vi "file header.vi"(8 "error in (no error)":errorcluster, 11 "Keywords Log File in":refnum<class "Keywords Log File.lvclass">) -> (0 "error out":errorcluster, 3 "Keywords Log File out":refnum<class "Keywords Log File.lvclass">)   [LabVIEW 2018, in "Keywords Log File.lvclass"]
uses:
  Keywords Log File.lvclass
  Log File/Log File.lvclass
  C:/Users/Denis/Desktop/S4ACS/S4ACS/Log File/Log File.lvclass
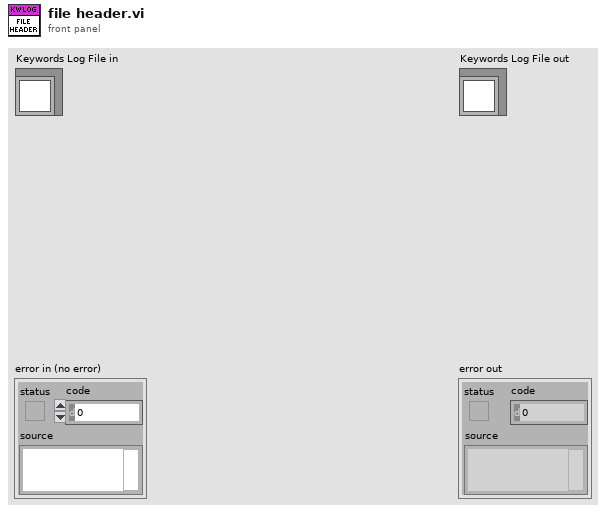
[diagram p1: front panel]
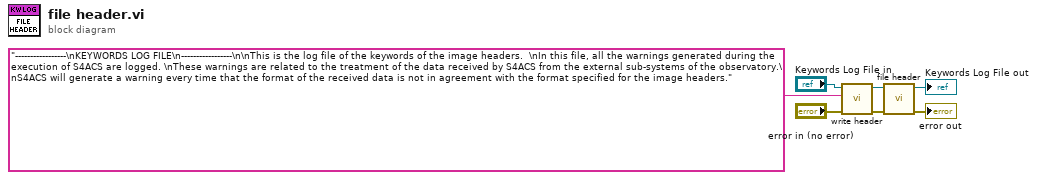
[diagram p0: block diagram]
diagram:
  n1 = call "write header.vi"("error in (no error)"="error in (no error)", "header"="-----------------\nKEYWORDS LOG FILE\n-----------------\n\nThis is the log file of the keywords of the image headers.  \nIn this file, all the warnings generated during the execution of S4ACS are logged. \nThese warnings are related to the treatment of the data received by S4ACS from the external sub-systems of the observatory.\nS4ACS will generate a warning every time that the format of the received data is not in agreement with the format specified for the image headers." ("message of the file header"), "Log File in"="Keywords Log File in") -> ("error out"=w5:errorcluster, "Log File out"=w4:refnum<class "Keywords Log File.lvclass">)  [unwired: 7 in]
  n2 = call-parent "file header.vi"("error in (no error)"=w5, "Log File in"=w4) -> ("error out"=→"error out":errorcluster, "Log File out"=→"Keywords Log File out":refnum<class "Keywords Log File.lvclass">)  [unwired: 8 in]
